vi "ex6-4.vi"   [LabVIEW 2013]
uses:
  <vilib>/NXT/Dual Mode Library/Sensors/EV3_Ultrasonic_CM.vi
  <vilib>/NXT/Dual Mode Library/Display/drawNumber_float.vi
  <vilib>/NXT/Dual Mode Library/Sensors/Touch_Pressed.vi
  <vilib>/NXT/NXTIO Xnodes/NXTIONodeSubVIs/LEGOStopAllMotors.vi
  <vilib>/NXT/NXTIO Xnodes/NXTIONodeSubVIs/LEGOMoveAllMotors.vi
  <vilib>/NXT/Subs/LVHSConnector.ctl
  <vilib>/NXT/NXTIO Xnodes/NXTIOXNode/NXTIO.xnode
  <vilib>/NXT/LegoClasses/BrickReference/BrickReference.lvclass
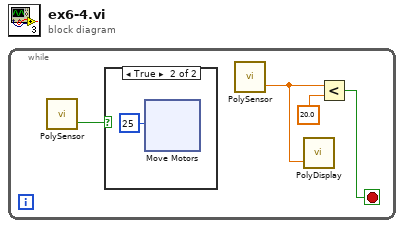
[diagram p0: block diagram]
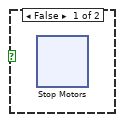
[diagram p2: hidden frame]
diagram:
  n1 = while {
    stop <- w3 stop-if-true
    n2 = call-poly <vilib>:"PolySensor.vi"() -> ("Yes / No"=w2:bool)  [unwired: 3 in, 1 out]
    n3 = case shown="True" w2 {
      frame False {
        n4 = xnode "Stop Motors"() -> ()  [unwired: 2 in, 1 out]
      }
      frame True {
        n5 = xnode "Move Motors"("Power/Speed 1"=i8 25) -> ()  [unwired: 2 in, 1 out]
      }
    }
    n6 = call-poly <vilib>:"PolySensor.vi"() -> ("Centimeters"=w1:sgl)  [unwired: 3 in, 1 out]
    n7 = call-poly <vilib>:"PolyDisplay.vi"("number"=w1) -> ()  [unwired: 3 in, 1 out]
    n8 = Less?(x=w1, y=sgl 20.0) -> (x < y?=w3:bool)
  }
